vi "Create.vi"(8 "error in (no error)":errorcluster, 11 "TopLevel in":refnum<class "GIS Printer.lvclass">) -> (0 "error out":errorcluster, 3 "TopLevel out":refnum<class "GIS Printer.lvclass">)   [LabVIEW 2022 SP3, in "GIS Printer.lvclass"]
uses:
  GIS Printer.lvclass
  GIS Printer.lvclass/GIS Printer.ctl
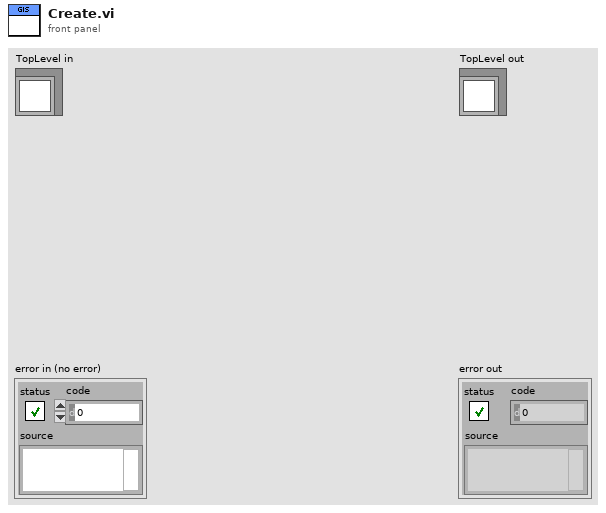
[diagram p1: front panel]
types:
  T1 = typedef "GIS Printer.lvclass/Private Data.ctl" = cluster{"UserEvents":T2, "All Dependencies":cluster{"Class References":refnum<class>[], "Class Names":string[]}, "PrinterConiguration":T3, "Status":T4, "GISHeadStatus":T5[], "HeadStatus":T6}
  T2 = typedef "GIS Printer.lvclass/UserEvents.ctl" = cluster{"API Incoming Event":refnum<user-event>, "API Executed Event":refnum<user-event>, "API Return Event":refnum<user-event>, "Status Changed Event":refnum<user-event>, "Abort":refnum<user-event>, "stop process":refnum<user-event>, "GISPollStatus":refnum<user-event>, "GISHeadStatus":refnum<user-event>, "Error Event":refnum<user-event>}
  T3 = typedef "GIS Printer.lvclass/PrinterConfiguration--Cluster.ctl" = cluster{"IPAddress":string, "Move Stage on RTP Command?":bool, "Stage Move Position":string, "PH1-Prime Path":path, "PH2-Prime Path":path, "PH3-Prime Path":path, "PH4-Prime Path":path, "PH5-Prime Path":path, "PH6-Prime Path":path, "PrintScriptsFolder":path, "PurgeScriptsFolder":path, "StageScriptsFolder":path, "PH1-HeatOn Path":path, "PH2-HeatOn Path":path, "PH3-HeatOn Path":path, "PH4-HeatOn Path":path, "PH5-HeatOn Path":path, "PH6-HeatOn Path":path, "PH1-HeatOff Path":path, "PH2-HeatOff Path":path, "PH3-HeatOff Path":path, "PH4-HeatOff Path":path, "PH5-HeatOff Path":path, "PH6-HeatOff Path":path}
  T4 = typedef "GIS Printer.lvclass/Status Cluster.ctl" = cluster{"Command Status":variant, "TCP Commands & Responses":string[][], "Printer Busy?":bool}
  T5 = typedef "GIS Status--Cluster.ctl" = cluster{"HeadEnabled":bool, "SpitEnabled":bool, "HeaterEnabled":bool, "TargetTemperature":dbl, "CurrentTemperature":dbl}
  T6 = typedef "HeadEnableStatus--cluster.ctl" = cluster{"PH1_Enable":bool, "PH2_Enable":bool, "PH3_Enable":bool, "PH4_Enable":bool, "PH5_Enable":bool, "PH6_Enable":bool}
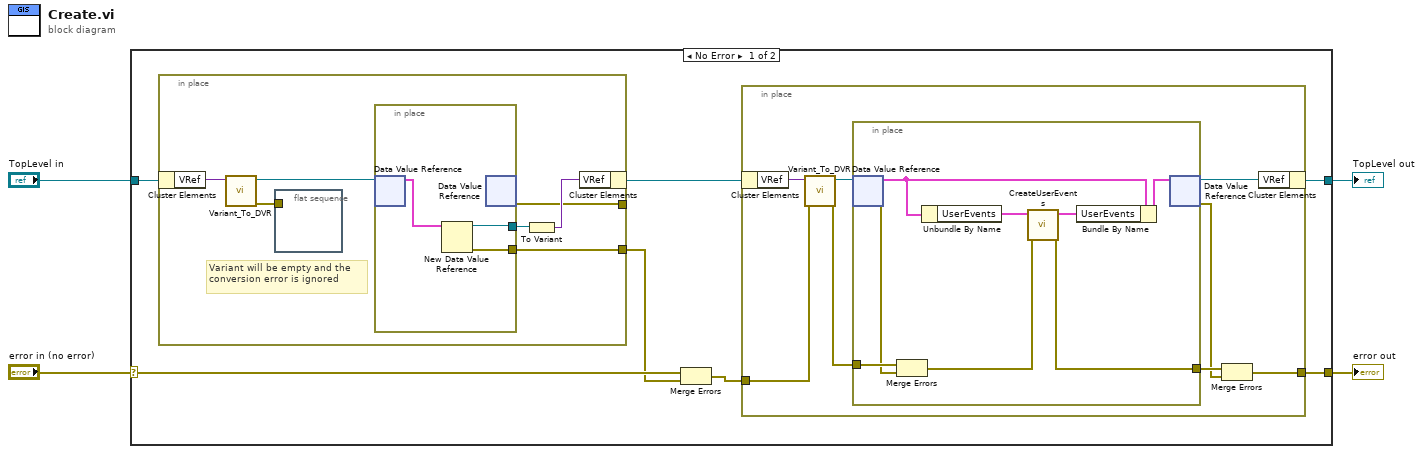
[diagram p0: block diagram]
diagram:
  n1 = case shown="No Error" "error in (no error)" {
    selector: "error in (no error)" -> [w11 w39]
    tunnel: [w5 w39] -> w3
    tunnel: [w7 w38] -> w1
    tunnel: "TopLevel in" -> [w10 w38]
    frame No Error {
      n2 = in-place {
        in-place-border: [w29] -> _
        in-place-border: [w28] -> w9
        # "Variant will be empty and the conversion error is ignored"
        n3 = in-place-cluster #1(w10) -> ("VRef"=w34:variant)
        n4 = call "Variant_To_DVR.vi"("Variant"=w34) -> ("error out"=w33:errorcluster, "DVR"=w32:refnum<data-value>)  [unwired: 9 in]
        n5 = flat-sequence {
          tunnel: w33 -> [_]
          frame #0 {
          }
        }
        n6 = in-place {
          in-place-border: [w36] -> w31
          in-place-border: [w35] -> w28
          n7 = in-place-dvr #2(w32) -> (w37:T1)  [unwired: 1 out]
          n8 = New Data Value Reference(data value=w37) -> (data value reference=w36:refnum<data-value>, error out=w35:errorcluster)  [unwired: 1 in]
          n9 = in-place-dvr #2() -> (w29:errorcluster)  [unwired: 1 in, 1 out]
        }
        n10 = To Variant(anything=w31) -> (Variant=w30:variant)
        n11 = in-place-cluster #1("VRef"=w30) -> (w8:refnum<class "GIS Printer.lvclass">)
      }
      n12 = Merge Errors(w11, w9) -> (w6:errorcluster)
      n13 = in-place {
        in-place-border: w6 -> [w17]
        in-place-border: [w13] -> w5
        n14 = in-place-cluster #3(w8) -> ("VRef"=w19:variant)
        n15 = call "Variant_To_DVR.vi"("error in (no error)"=w17, "Variant"=w19) -> ("error out"=w16:errorcluster, "DVR"=w18:refnum<data-value>)  [unwired: 8 in]
        n16 = in-place {
          in-place-border: w16 -> [w23]
          in-place-border: [w20] -> w15
          n17 = in-place-dvr #4(w18) -> (w26:T1, w21:errorcluster)
          n18 = Merge Errors(w23, w21) -> (w22:errorcluster)
          n19 = Unbundle By Name(w26) -> ("UserEvents"=w27:T2)
          n20 = call "CreateUserEvents.vi"("error in (no error)"=w22, "UserEvents"=w27) -> ("error out"=w20:errorcluster, "UserEvents out"=w25:T2)  [unwired: 8 in]
          n21 = Bundle By Name(cluster=w26, "UserEvents"=w25) -> (w24:T1)
          n22 = in-place-dvr #4(w24) -> (w12:refnum<data-value>, w14:errorcluster)
        }
        n23 = Merge Errors(w15, w14) -> (w13:errorcluster)
        n24 = in-place-cluster #3("VRef"=w12) -> (w7:refnum<class "GIS Printer.lvclass">)
      }
    }
    frame Error {
    }
  }
  "error out" <- w3
  "TopLevel out" <- w1
